vi "Is Valid File.vi"(8 "Error In":errorcluster, 11 "File":path) -> (0 "Error Out":errorcluster, 2 "Valid file":bool, 3 "File out":path)   [LabVIEW 2015]
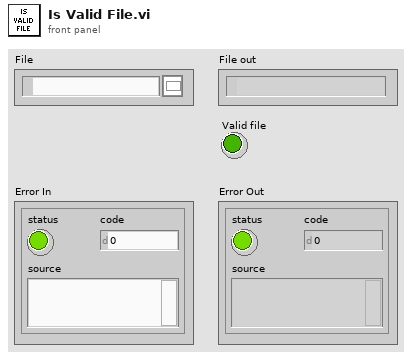
[diagram p1: front panel]
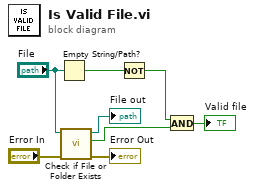
[diagram p0: block diagram]
diagram:
  n1 = Empty String/Path?(string/path="File") -> (empty?=w6:bool)
  n2 = call <vilib>:"Check if File or Folder Exists.vi"("error in (no error)"="Error In", "path"="File") -> ("error out"=→"Error Out":errorcluster, "file or folder exists?"=w8:bool, "dup path"=→"File out":path)  [unwired: 7 in]
  n3 = Not(x=w6) -> (.not. x?=w7:bool)
  n4 = And(x=w7, y=w8) -> (x .and. y?=→"Valid file":bool)
